vi "exercicios6_string.vi"() -> ()   [LabVIEW 2018]
panel:
  out "s? t:f":string
  in  "String":string
  out "2291,111233 to number":dbl
  out "233 to number":i32
  out "12,998821 to string":string
  out "4556 to string":string
  out "concatenated string":string
  in  "string":string
  # "Exercício 1"
  # "Exercício 2"
  # "Exercício 3"
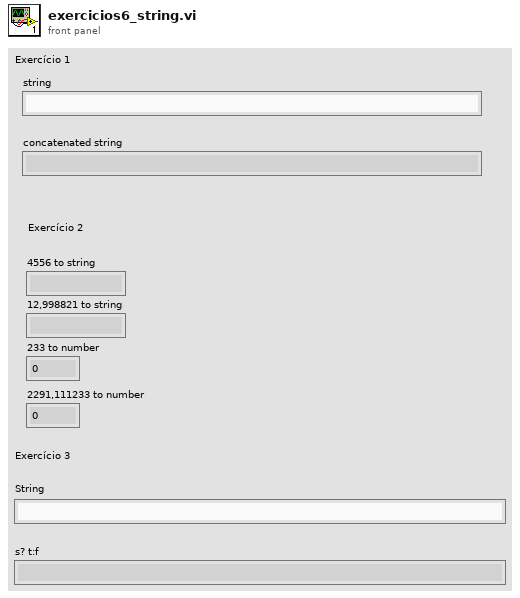
[diagram p1: front panel]
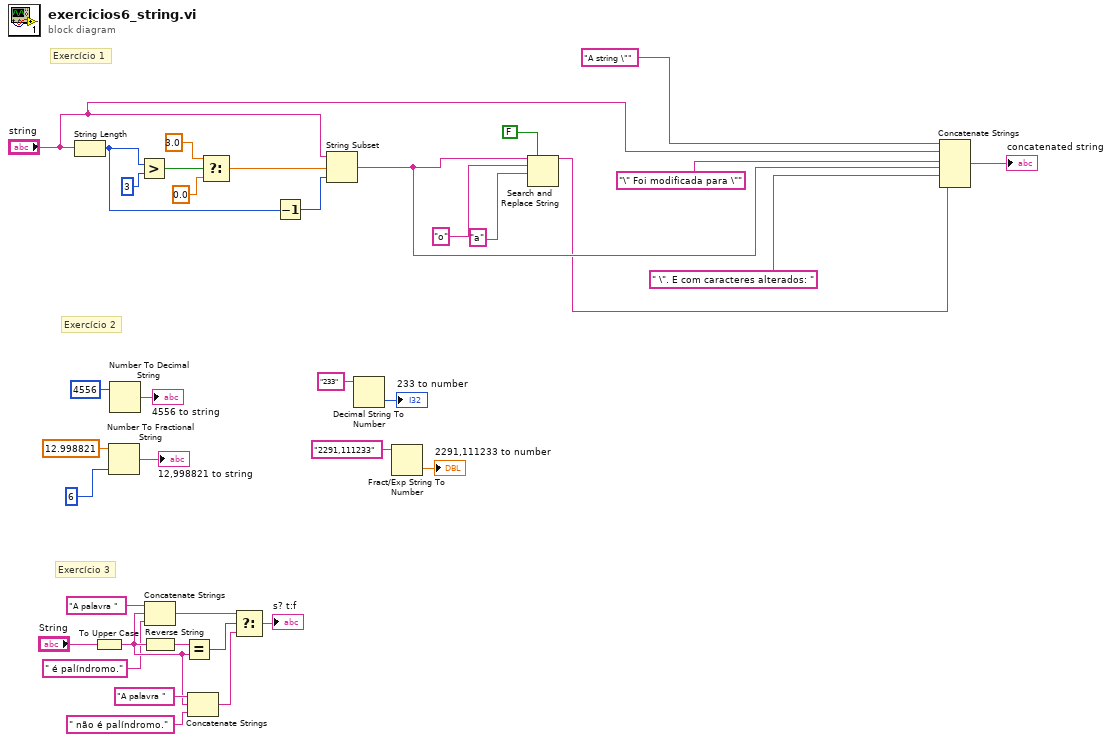
[diagram p0: block diagram]
diagram:
  # "Exercício 3"
  # "Exercício 2"
  # "Exercício 1"
  n1 = String Length(string="string") -> (length=w32:i32)
  n2 = To Upper Case(1:"String") -> (0:w6:string)
  n3 = Number To Fractional String(number=12.998821, precision (6)=i16 6) -> (F-format string=→"12,998821 to string":string)  [unwired: 2 in]
  n4 = Number To Decimal String(number=4556) -> (decimal integer string=→"4556 to string":string)  [unwired: 1 in]
  n5 = Greater?(x=w32, y=3) -> (0:w36:bool)
  n6 = Concatenate Strings("A palavra " ("string"), w6, " é palíndromo." ("string")) -> (w2:string)
  n7 = Reverse String(1:w6) -> (0:w10:string)
  n8 = Equal?(x=w10, y=w6) -> (x = y?=w9:bool)
  n9 = Concatenate Strings("A palavra " ("string"), w6, " não é palíndromo." ("string")) -> (w4:string)
  n10 = Select(t=3.0, s=w36, f=0.0) -> (s? t:f=w33:dbl)
  n11 = Select(t=w2, s=w9, f=w4) -> (s? t:f=→"s? t:f":string)
  n12 = Decrement(x=w32) -> (x-1=w31:i32)
  n13 = String Subset(string="string", offset (0)=w33, length (rest)=w31) -> (substring=w24:string)
  n14 = Decimal String To Number(string="233") -> (number=→"233 to number":i32)  [unwired: 2 in, 1 out]
  n15 = Fract/Exp String To Number(string="2291,111233") -> (number=→"2291,111233 to number":dbl)  [unwired: 3 in, 1 out]
  n16 = Search and Replace String(replace all?=FALSE ("replace all? (F)"), input string=w24, search string="o", replace string="a" ("replace string (\"\")")) -> (result string=w21:string)  [unwired: 4 in, 3 out]
  n17 = Concatenate Strings("A string \"" ("string"), "string", "\" Foi modificada para \"" ("string"), w24, " \". E com caracteres alterados: " ("string"), w21) -> (→"concatenated string":string)
